vi "Read Test Case.lvclass.vi"(8 "error in (no error)":errorcluster, 11 "Class 1 in":refnum<class "Class 1.lvclass">) -> (0 "error out":errorcluster, 2 "Test Case.lvclass":refnum<class "Test Case.lvclass">, 3 "Class 1 out":refnum<class "Class 1.lvclass">)   [LabVIEW 2020, in "Class 1.lvclass"]
uses:
  Class 1.lvclass
  <vilib>/Astemes/LUnit/Test Case.lvclass
  Class 1.lvclass/Class 1.ctl
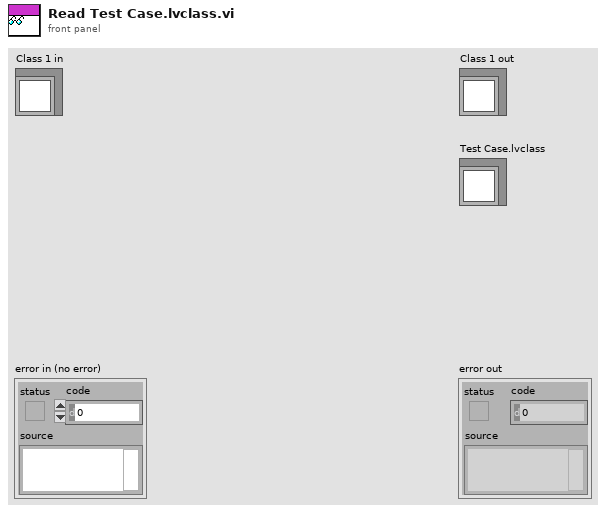
[diagram p1: front panel]
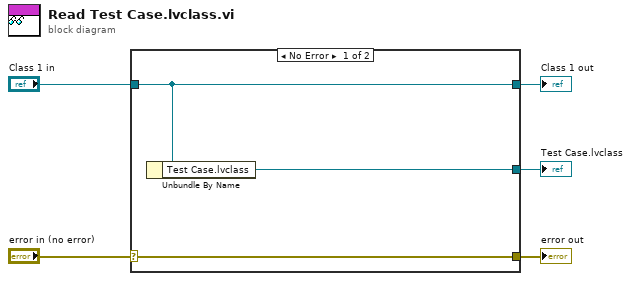
[diagram p0: block diagram]
diagram:
  n1 = case shown="No Error" "error in (no error)" {
    selector: "error in (no error)" -> [w8 w9]
    tunnel: [w8 w9] -> w4
    tunnel: [w7 w10] -> w2
    tunnel: "Class 1 in" -> [w7 w10]
    tunnel: [w6 _] -> w1
    frame No Error {
      n2 = Unbundle By Name(w7) -> ("Test Case.lvclass"=w6:refnum<class "Test Case.lvclass">)
    }
    frame Error {
    }
  }
  "error out" <- w4
  "Class 1 out" <- w2
  "Test Case.lvclass" <- w1
